vi "GetFailures.vi"(8 "error in (no error)":errorcluster, 11 "TestResult in":refnum<class "TestResult.lvclass">) -> (0 "error out":errorcluster, 2 "failures":T1[](array[typedef]), 3 "TestResult out":refnum<class "TestResult.lvclass">)   [LabVIEW 2013, in "TestResult.lvclass"]
uses:
  TestResult.lvclass
  private/failure.ctl
  TestResult.lvclass/TestResult.ctl
panel:
  # "JKI VI Tester for LabVIEW\nhttp://jkisoft.com/vi-tester\nCopyright (C) 2007-2009, JKI <info@jkisoft.com>\nALL RIGHTS RESERVED"
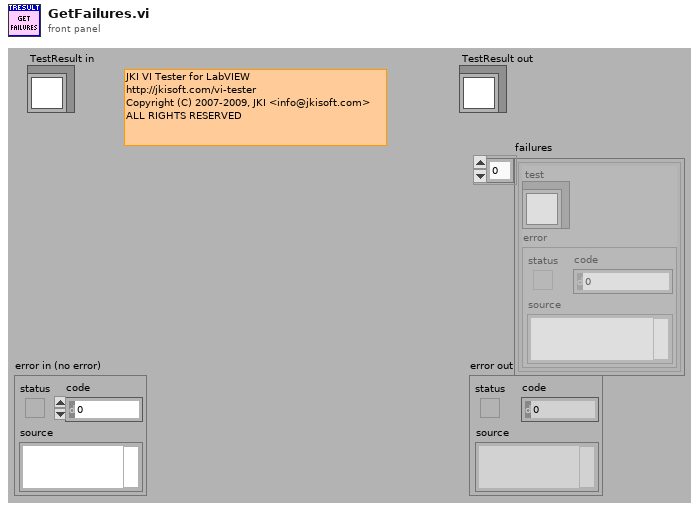
[diagram p1: front panel]
types:
  T1 = typedef "TestResult.lvclass/failure.ctl" = cluster{"test":refnum<class>, "error":errorcluster}
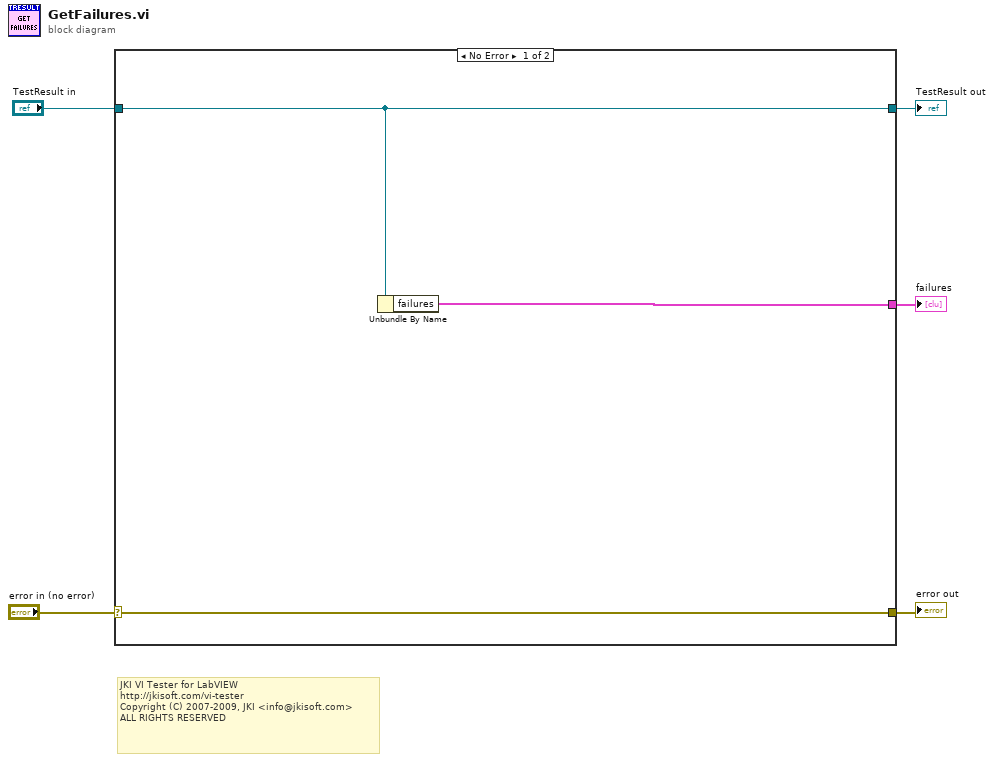
[diagram p0: block diagram]
diagram:
  # "JKI VI Tester for LabVIEW\nhttp://jkisoft.com/vi-tester\nCopyright (C) 2007-2009, JKI <info@jkisoft.com>\nALL RIGHTS RESERVED"
  n1 = case shown="No Error" "error in (no error)" {
    selector: "error in (no error)" -> [w7 w10]
    tunnel: [w7 w10] -> w4
    tunnel: [w6 w9] -> w2
    tunnel: "TestResult in" -> [w6 w9]
    tunnel: [w8 _] -> w1
    frame No Error {
      n2 = Unbundle By Name(w6) -> ("failures"=w8:T1[])
    }
    frame Error {
    }
  }
  "error out" <- w4
  "TestResult out" <- w2
  "failures" <- w1
